vi "摆角标度变换-子.vi"(3 "摆角输入":dbl) -> (0 "布尔":bool, 1 "摆角输出":dbl)   [LabVIEW 2015]
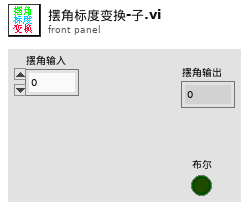
[diagram p1: front panel]
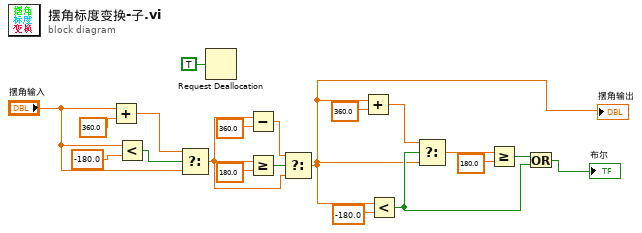
[diagram p0: block diagram]
diagram:
  n1 = Add(x="摆角输入", y=360.0) -> (x+y=w17:dbl)
  n2 = Less?(x="摆角输入", y=-180.0) -> (x < y?=w19:bool)
  n3 = Select(t=w17, s=w19, f="摆角输入") -> (s? t:f=w12:dbl)
  n4 = Request Deallocation(TRUE ("标志")) -> ()
  n5 = Subtract(x=w12, y=360.0) -> (x-y=w13:dbl)
  n6 = Greater Or Equal?(x=w12, y=180.0) -> (x >= y?=w16:bool)
  n7 = Select(t=w13, s=w16, f=w12) -> (s? t:f=w3:dbl)
  "摆角输出" <- w3
  n8 = Add(x=w3, y=360.0) -> (x+y=w9:dbl)
  n9 = Less?(x=w3, y=-180.0) -> (x < y?=w5:bool)
  n10 = Select(t=w9, s=w5, f=w3) -> (s? t:f=w7:dbl)
  n11 = Greater Or Equal?(x=w7, y=180.0) -> (x >= y?=w6:bool)
  n12 = Or(x=w6, y=w5) -> (x .or. y?=→"布尔":bool)
